vi "Destroy_ErrorHandler.vi"(8 "error in (no error)":errorcluster, 11 "ErrorHandler in":refnum<class "ErrorHandler.lvclass">) -> (0 "error out":errorcluster, 3 "ErrorHandler out":refnum<class "ErrorHandler.lvclass">)   [LabVIEW 2019, in "ErrorHandler.lvclass"]
doc: "Developed by Kevin Thompson\nkevin@thompsonengineering.net\n\nCopyright 2018\nThompson Engineering, LLC"
uses:
  ErrorHandler.lvclass
  TypeDef/TD GetSet ActionSelect--enum.ctl
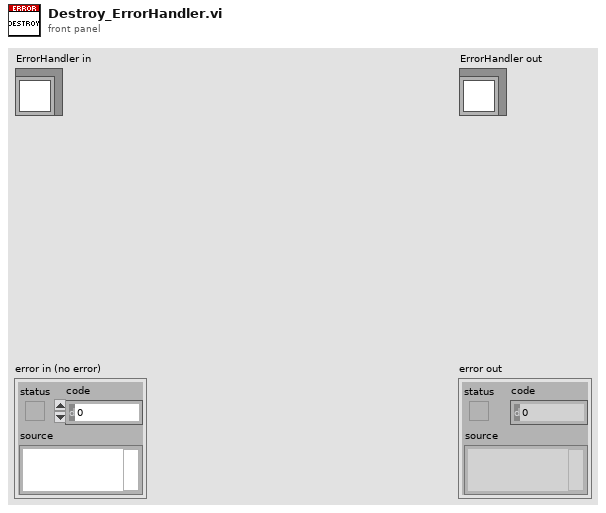
[diagram p1: front panel]
types:
  T1 = typedef "ErrorHandler.lvclass/TD GetSet ActionSelect--enum.ctl" = enum16{"Init", "Get", "Set"}
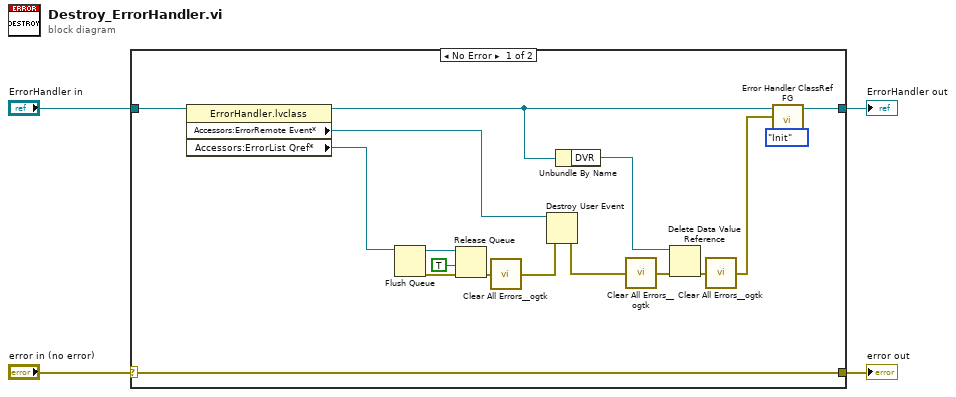
[diagram p0: block diagram]
diagram:
  n1 = case shown="No Error" "error in (no error)" {
    selector: "error in (no error)" -> [w21 w23]
    tunnel: [w21 w23] -> w3
    tunnel: [w11 w22] -> w1
    tunnel: "ErrorHandler in" -> [w7 w22]
    frame No Error {
      n2 = property class="ErrorHandler.lvclass"(reference=w7) -> (reference out=w8:refnum<class "ErrorHandler.lvclass">, "Accessors:ErrorRemote Event*"=w6:refnum<user-event>, "Accessors:ErrorList Qref*"=w5:refnum<queue>)  [unwired: 1 in, 1 out]
      n3 = Flush Queue(queue=w5) -> (queue out=w20:refnum<queue>, error out=w19:errorcluster)  [unwired: 1 in, 1 out]
      n4 = Release Queue(queue=w20, force destroy? (F)=TRUE, error in (no error)=w19) -> (error out=w16:errorcluster)  [unwired: 2 out]
      n5 = call <userlib>:"Clear All Errors__ogtk.vi"("Error In"=w16) -> ("Error Out"=w15:errorcluster)  [unwired: 3 in]
      n6 = Destroy User Event(user event=w6, error in=w15) -> (error out=w14:errorcluster)
      n7 = Unbundle By Name(w8) -> ("DVR"=w17:refnum<data-value>)
      n8 = call <userlib>:"Clear All Errors__ogtk.vi"("Error In"=w14) -> ("Error Out"=w13:errorcluster)  [unwired: 3 in]
      n9 = Delete Data Value Reference(data value reference=w17, error in=w13) -> (error out=w10:errorcluster)  [unwired: 1 out]
      n10 = call <userlib>:"Clear All Errors__ogtk.vi"("Error In"=w10) -> ("Error Out"=w9:errorcluster)  [unwired: 3 in]
      n11 = call "Error Handler ClassRef FG.vi"("action (Get)"=TD_GetSet_ActionSelect--enum."Init", "error in (no error)"=w9, "ErrorHandler in"=w8) -> ("ErrorHandler out"=w11:refnum<class "ErrorHandler.lvclass">)  [unwired: 7 in, 1 out]
    }
    frame Error {
    }
  }
  "error out" <- w3
  "ErrorHandler out" <- w1
